vi "Angle Set.vi"(9 "Set Angle?":bool, 10 "Angle Set":dbl, 11 "Angle In":dbl) -> (3 "New Angle Out":dbl)   [LabVIEW 2015]
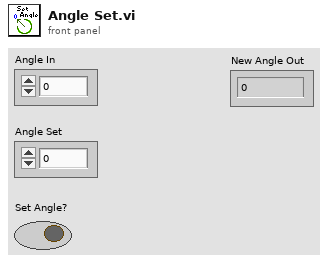
[diagram p1: front panel]
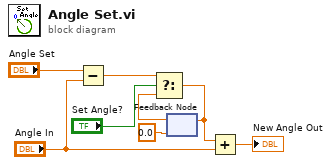
[diagram p0: block diagram]
diagram:
  n1 = Subtract(x="Angle Set", y="Angle In") -> (x-y=w5:dbl)
  n2 = feedback #1(0.0) -> (w4:dbl)
  n3 = Select(t=w5, s="Set Angle?", f=w4) -> (s? t:f=w3:dbl)
  n4 = feedback-in #1(w3) -> ()
  n5 = Add(x=w3, y="Angle In") -> (x+y=→"New Angle Out":dbl)
